vi "Resolve DB Bin File Name and Path.vi"(8 "error in":errorcluster, 11 "DB XML File":path) -> (0 "error out":errorcluster, 1 "SysExec":string, 2 "Destination File":path, 3 "Converted File":path)   [LabVIEW 2011, in "AIT 429 Custom Device.lvlib"]
uses:
  AIT 429 Custom Device.lvlib
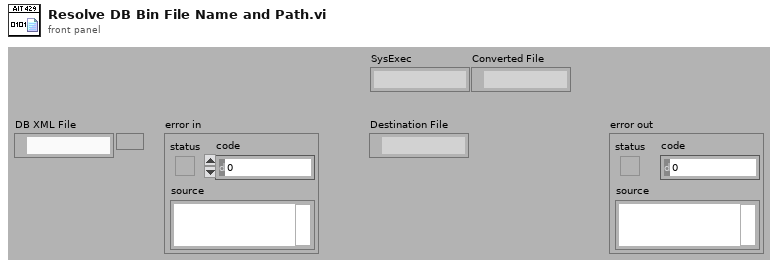
[diagram p1: front panel]
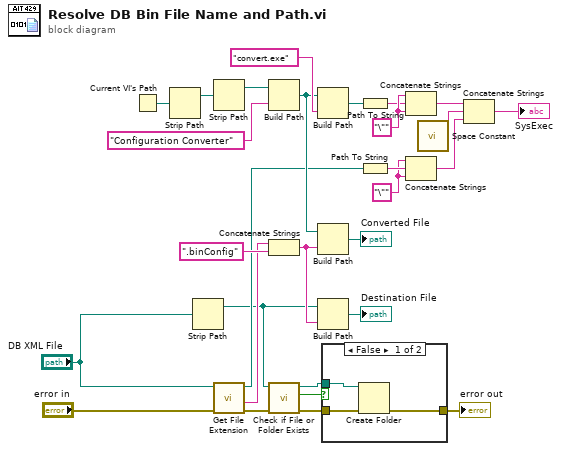
[diagram p0: block diagram]
diagram:
  w16 = "\"" ("string")
  w20 = "\"" ("string")
  n1 = Current VI's Path() -> (path=w25:path)
  n2 = Strip Path(path=w25) -> (stripped path=w24:path)  [unwired: 1 out]
  n3 = Strip Path(path="DB XML File") -> (stripped path=w2:path)  [unwired: 1 out]
  n4 = Strip Path(path=w24) -> (stripped path=w23:path)  [unwired: 1 out]
  n5 = call <vilib>:"Get File Extension.vi"("error in (no error)"="error in", "file"="DB XML File") -> ("error out"=w7:errorcluster, "filename without extension"=w27:string, "dup file"=w8:path)  [unwired: 6 in, 1 out]
  n6 = Build Path(base path=w23, name or relative path="Configuration Converter") -> (appended path=w11:path)
  n7 = Concatenate Strings(w27, ".binConfig" ("string")) -> (w10:string)
  n8 = call <vilib>:"Check if File or Folder Exists.vi"("error in (no error)"=w7, "path"=w2) -> ("error out"=w4:errorcluster, "file or folder exists?"=w6:bool, "dup path"=w3:path)  [unwired: 7 in]
  n9 = Build Path(base path=w11, name or relative path="convert.exe") -> (appended path=w19:path)
  n10 = Build Path(base path=w11, name or relative path=w10) -> (appended path=→"Converted File":path)
  n11 = Build Path(base path=w2, name or relative path=w10) -> (appended path=→"Destination File":path)
  n12 = case shown="False" w6 {
    tunnel: [w30 w33] -> w5
    tunnel: w4 -> [w32 w33]
    tunnel: w3 -> [w31 _]
    frame False {
      n13 = Create Folder(path (use dialog)=w31, error in=w32) -> (error out=w30:errorcluster)  [unwired: 1 in, 2 out]
    }
    frame True {
    }
  }
  "error out" <- w5
  n14 = Path To String(path=w19) -> (string=w18:string)
  n15 = Path To String(path=w8) -> (string=w17:string)
  n16 = Concatenate Strings(w20, w18, w20) -> (w12:string)
  n17 = Concatenate Strings(w16, w17, w16) -> (w14:string)
  n18 = call <vilib>:"Space Constant.vi"() -> ("String"=w15:string)
  n19 = Concatenate Strings(w12, w15, w14) -> (→"SysExec":string)
